vi "Validate CFG.vi"(8 "Error In":errorcluster, 11 "<JSON>":string) -> (0 "Error Out":errorcluster, 2 "Is Valid?":bool)   [LabVIEW 2023, in "Configuration UI Actor.lvlib" / "Configuration UI Actor.lvclass"]
uses:
  Configuration UI Actor.lvclass
  Configuration UI Actor.lvclass/Configuration UI Actor.ctl
  <vilib>/Utility/error.llb/Error Cluster From Error Code.vi
  <vilib>/ErrorRing/Error Ring.xnode
  HAL GOOP4/Configuration JSON Base/CFG JSON Base.lvclass
  7f7e7bab-2ea2-4962-b1fc-52cde1125a58.vi
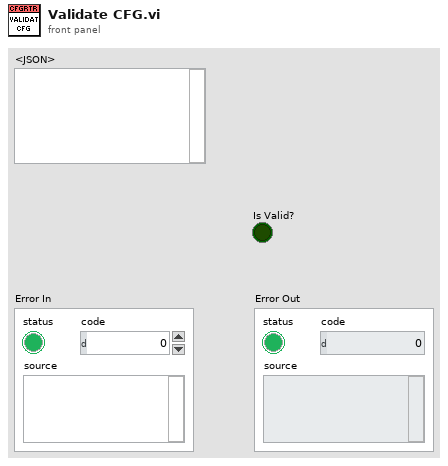
[diagram p1: front panel]
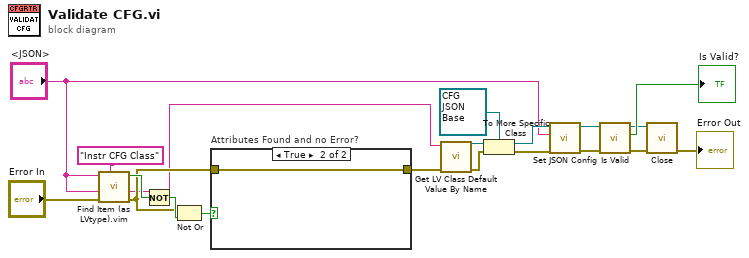
[diagram p0: block diagram]
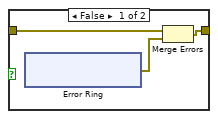
[diagram p2: hidden frame]
diagram:
  n1 = call "Find Item (as LVtype).vim"("$Path or Item Name"="Instr CFG Class", "error in (no error)"="Error In", "Data Type and Default Value"="<JSON>", "JSON"="<JSON>") -> ("error out"=w16:errorcluster, "Data"=w11:string, "Found"=w18:bool)  [unwired: 4 in, 1 out]
  n2 = Not(x=w18) -> (.not. x?=w20:bool)
  n3 = Not Or(1:w20, 2:w16) -> (0:w19:bool)
  n4 = case "Attributes Found and no Error?" shown="True" w19 {
    tunnel: [w23 w29] -> w17
    tunnel: w16 -> [w21 w29]
    frame False {
      n5 = xnode "Error Ring"() -> ("error out"=w22:errorcluster)
      n6 = Merge Errors(w21, w22) -> (w23:errorcluster)
    }
    frame True {
    }
  }
  n7 = call <vilib>:"Get LV Class Default Value By Name.vi"("error in (no error)"=w17, "class name"=w11) -> ("error out"=w14:errorcluster, "object"=w13:refnum<class>)  [unwired: 8 in]
  n8 = To More Specific Class(target class=refnum<class "CFG JSON Base.lvclass"> refnum ("HAL GOOP4.lvlib:CFG JSON Base.lvclass"), reference=w13, error in=w14) -> (specific class reference=w10:refnum<class "CFG JSON Base.lvclass">, error out=w9:errorcluster)
  n9 = call "Set JSON Config.vi"("error in (no error)"=w9, "<JSON>Config>"="<JSON>", "CFG Base in"=w10) -> ("error out"=w6:errorcluster, "CFG Base out"=w7:refnum<class "CFG JSON Base.lvclass">)  [unwired: 7 in]
  n10 = call-dynamic "Is Valid.vi"("error in (no error)"=w6, "CFG JSON Base in"=w7) -> ("error out"=w3:errorcluster, "Is Valid?"=→"Is Valid?":bool, "CFG JSON Base out"=w2:refnum<class "CFG JSON Base.lvclass">)  [unwired: 7 in]
  n11 = call-dynamic "Close.vi"("error in (no error)"=w3, "IConfigure in"=w2) -> ("error out"=→"Error Out":errorcluster)  [unwired: 8 in, 1 out]
